vi "Freq_Positive.vi"(0 "enter freq [MHz]":dbl format="%.2f") -> (1 "T1 command  str":string, 2 "T2 command  str":string, 3 "T3 command  str":string)   [LabVIEW 2022 SP3]
panel:
  out "T3":i16
  out "HEX":string
  out "T2":i16
  out "HEX":string
  out "HEX":string
  out "period in steps":i32
  out "T1":i16
  out "period [nSec]":dbl format="%.2f"
  # "HIGH"
  # "DEAD"
  # "LOW"
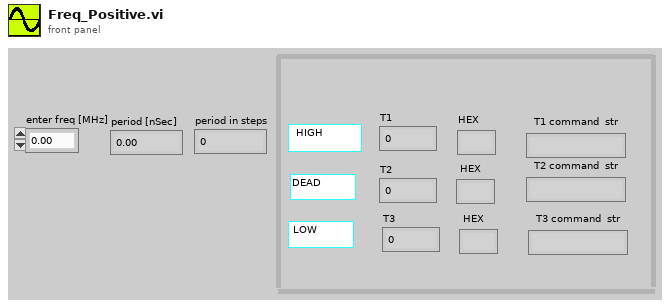
[diagram p1: front panel]
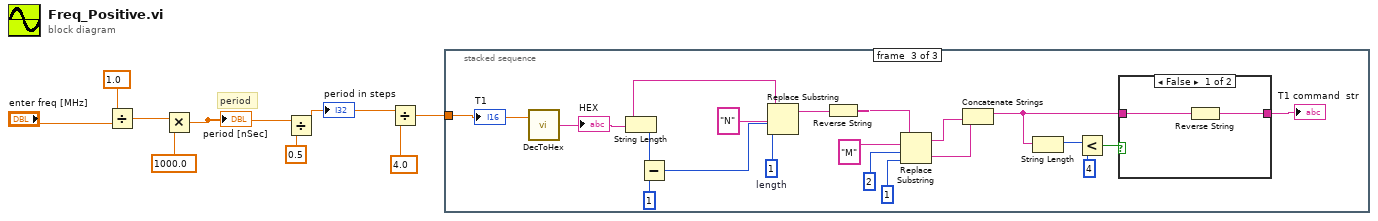
[diagram p0: block diagram]
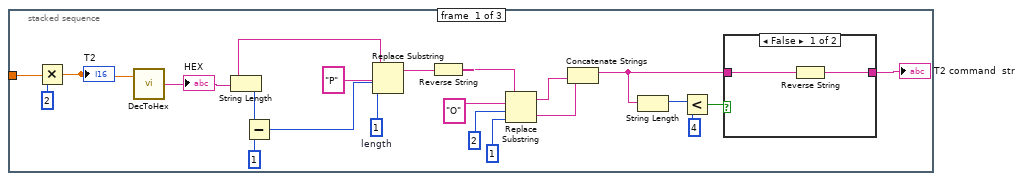
[diagram p2: hidden frame]
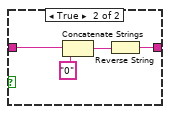
[diagram p3: hidden frame]
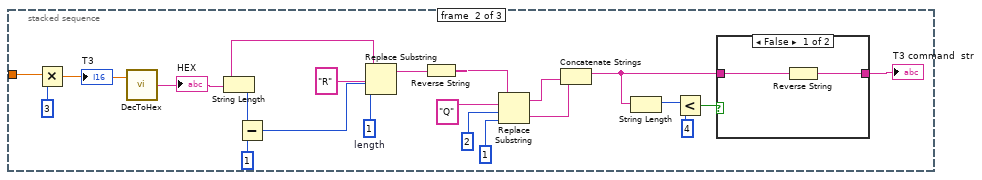
[diagram p4: hidden frame]
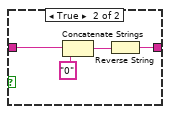
[diagram p5: hidden frame]
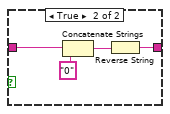
[diagram p6: hidden frame]
diagram:
  # "period"
  n1 = Divide(x=1.0, y="enter freq [MHz]") -> (x/y=w4:dbl)
  n2 = Multiply(x=w4, y=1000.0) -> (x*y=w5:dbl)
  "period [nSec]" <- w5
  n3 = Divide(x=w5, y=0.5) -> (x/y=w2:dbl)
  "period in steps" <- w2
  n4 = Divide(x=w2, y=4.0) -> (x/y=w1:dbl)
  n5 = stacked-sequence {
    tunnel: w1 -> [w10 w37 w65]
    frame #0 {
      w29 = 1  # length
      n6 = Multiply(x=w10, y=2) -> (x*y=w11:dbl)
      "T2" <- w11
      n7 = call "DecToHex.vi"("Decimal . Decimal Representation"=w11) -> ("HEX . HEX representation"=w12:string)  [unwired: 1 out]
      "HEX" <- w12
      n8 = String Length(string=w12) -> (length=w27:i32)
      n9 = Subtract(x=w27, y=1) -> (x-y=w15:i32)
      n10 = Replace Substring(2:w29, 3:w15, 4:"P", 5:w12) -> (1:w26:string)  [unwired: 1 out]
      n11 = Reverse String(1:w26) -> (0:w25:string)
      n12 = Replace Substring(2:1, 3:2, 4:"O", 5:w25) -> (0:w20:string, 1:w21:string)
      n13 = Concatenate Strings(w21, w20) -> (w17:string)
      n14 = String Length(string=w17) -> (length=w19:i32)
      n15 = Less?(x=w19, y=4) -> (x < y?=w16:bool)
      n16 = case shown="False" w16 {
        tunnel: w17 -> [w32 w35]
        tunnel: [w31 w33] -> w13
        frame False {
          n17 = Reverse String(1:w32) -> (0:w31:string)
        }
        frame True {
          n18 = Concatenate Strings(w35, "0") -> (w34:string)
          n19 = Reverse String(1:w34) -> (0:w33:string)
        }
      }
      "T2 command  str" <- w13
    }
    frame #1 {
      w56 = 1  # length
      n20 = Multiply(x=w37, y=3) -> (x*y=w38:dbl)
      "T3" <- w38
      n21 = call "DecToHex.vi"("Decimal . Decimal Representation"=w38) -> ("HEX . HEX representation"=w39:string)  [unwired: 1 out]
      "HEX" <- w39
      n22 = String Length(string=w39) -> (length=w54:i32)
      n23 = Subtract(x=w54, y=1) -> (x-y=w42:i32)
      n24 = Replace Substring(2:w56, 3:w42, 4:"R", 5:w39) -> (1:w53:string)  [unwired: 1 out]
      n25 = Reverse String(1:w53) -> (0:w52:string)
      n26 = Replace Substring(2:1, 3:2, 4:"Q", 5:w52) -> (0:w47:string, 1:w48:string)
      n27 = Concatenate Strings(w48, w47) -> (w44:string)
      n28 = String Length(string=w44) -> (length=w46:i32)
      n29 = Less?(x=w46, y=4) -> (x < y?=w43:bool)
      n30 = case shown="False" w43 {
        tunnel: w44 -> [w59 w62]
        tunnel: [w58 w60] -> w40
        frame False {
          n31 = Reverse String(1:w59) -> (0:w58:string)
        }
        frame True {
          n32 = Concatenate Strings(w62, "0") -> (w61:string)
          n33 = Reverse String(1:w61) -> (0:w60:string)
        }
      }
      "T3 command  str" <- w40
    }
    frame #2 {
      w82 = 1  # length
      n34 = call "DecToHex.vi"("Decimal . Decimal Representation"=w65) -> ("HEX . HEX representation"=w64:string)  [unwired: 1 out]
      "HEX" <- w64
      n35 = String Length(string=w64) -> (length=w80:i32)
      n36 = Subtract(x=w80, y=1) -> (x-y=w68:i32)
      n37 = Replace Substring(2:w82, 3:w68, 4:"N", 5:w64) -> (1:w79:string)  [unwired: 1 out]
      n38 = Reverse String(1:w79) -> (0:w78:string)
      n39 = Replace Substring(2:1, 3:2, 4:"M", 5:w78) -> (0:w73:string, 1:w74:string)
      n40 = Concatenate Strings(w74, w73) -> (w70:string)
      n41 = String Length(string=w70) -> (length=w72:i32)
      n42 = Less?(x=w72, y=4) -> (x < y?=w69:bool)
      n43 = case shown="False" w69 {
        tunnel: w70 -> [w84 w87]
        tunnel: [w83 w85] -> w66
        frame False {
          n44 = Reverse String(1:w84) -> (0:w83:string)
        }
        frame True {
          n45 = Concatenate Strings(w87, "0") -> (w86:string)
          n46 = Reverse String(1:w86) -> (0:w85:string)
        }
      }
      "T1 command  str" <- w66
      "T1" <- w65
    }
  }
